vi "PROIECT1.vi"() -> ()   [LabVIEW 2021]
uses:
  <vilib>/express/express arith-compare/Formula/XNode/ExpressFormulaBlockNode.xnode
panel:
  in  "stop":bool
  in  "Boolean":bool
  out "Waveform Chart":cluster{"Knob":dbl, "Result":dbl, "Knob":dbl}(graph)
  out "?":string
  in  "Knob 2":dbl(knob) scale=0.0..100.0
  in  "Dial":dbl(knob) scale=0.0..100.0
  in  "Knob":dbl(knob) scale=0.0..100.0
  out "KELVIN":dbl(slide) scale=0.0..400.0
  out "FARENHEIT":dbl(slide) scale=0.0..200.0
  out "CELSIUS":dbl(slide) scale=0.0..100.0
  out "nr. aleator":dbl format="%#_2g"
  out "Temp aleatoare":dbl format="%#_3g"
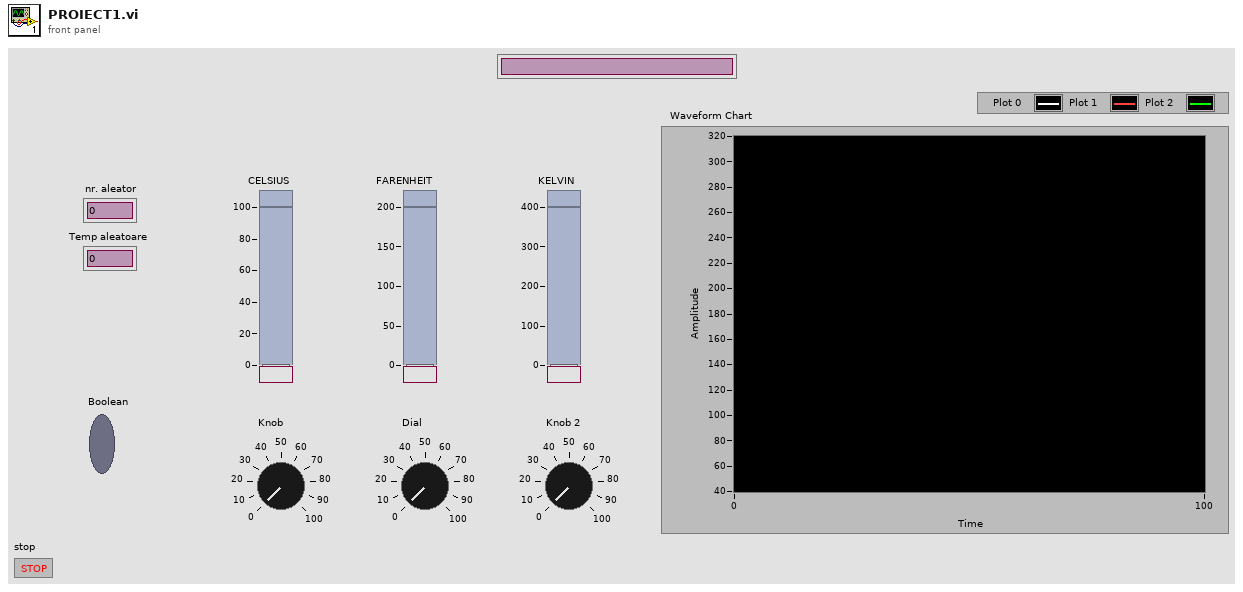
[diagram p1: front panel]
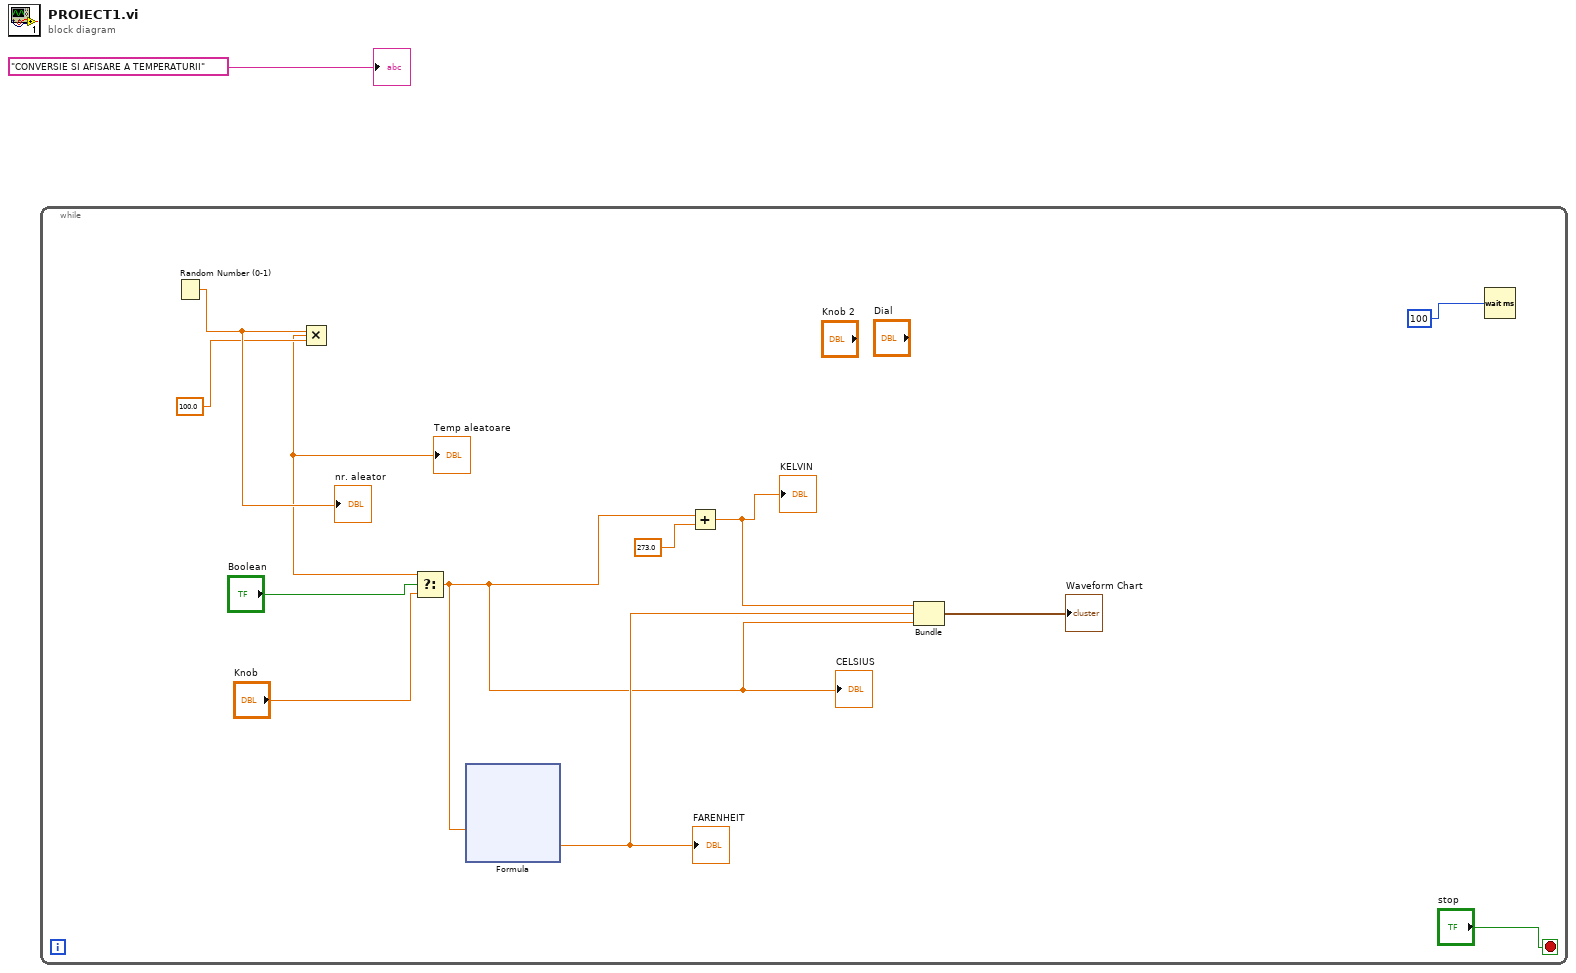
[diagram p0: block diagram]
diagram:
  n1 = while {
    stop <- "stop" stop-if-true
    n2 = Random Number (0-1)() -> (number: 0 to 1=w13:dbl)
    "nr. aleator" <- w13
    n3 = Multiply(x=w13, y=100.0 ("x")) -> (x*y=w11:dbl)
    "Temp aleatoare" <- w11
    n4 = Select(t=w11, s="Boolean", f="Knob") -> (s? t:f=w6:dbl)
    "CELSIUS" <- w6
    n5 = xnode "Formula"("X1"=w6) -> ("Result"=w7:dbl)  [unwired: 1 in, 1 out]
    "FARENHEIT" <- w7
    n6 = Add(x=w6, y=273.0) -> (x+y=w4:dbl)
    "KELVIN" <- w4
    n7 = Bundle(w4, "Result"=w7, "Knob"=w6) -> (→"Waveform Chart":cluster{dbl, "Result":dbl, "Knob":dbl})  [unwired: 1 in]
    n8 = Wait (ms)(milliseconds to wait=u32 100 ("millisecond timer value")) -> ()  [unwired: 1 out]
  }
  "?" <- "CONVERSIE SI AFISARE A TEMPERATURII" ("String")
